vi "Write Digital Port.vi"(8 "error in (no error)":errorcluster, 10 "DOs":bool[](array[boolean]), 11 "Digital Output in":refnum<class "Digital IO Instrument.lvclass">) -> (0 "error out":errorcluster, 3 "Digital Output out":refnum<class "Digital IO Instrument.lvclass">)   [LabVIEW 2025, in "Digital IO.lvlib" / "Digital IO Instrument.lvclass"]
uses:
  Digital IO Instrument.lvclass
  Digital IO Instrument.lvclass/Digital IO Instrument.ctl
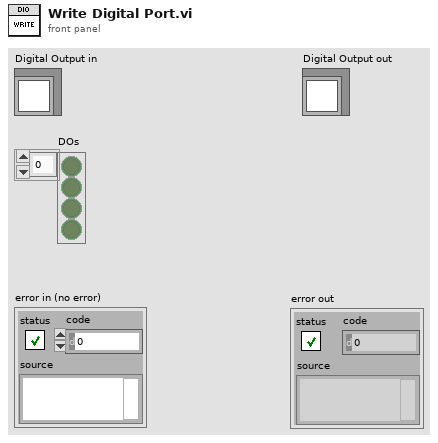
[diagram p1: front panel]
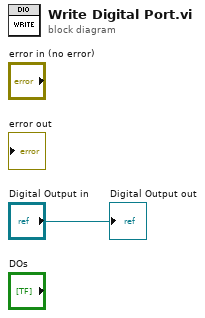
[diagram p0: block diagram]
diagram:
  "Digital Output out" <- "Digital Output in"
